vi "mtlb simx Call Script Function b.vi"(0 "clientID":i32, 1 "outString":string, 5 "variousIntsOut":i32, 7 "outInt":i32, 9 "outFloat":sgl, 11 "error in (no error)":errorcluster, 12 "outBuffer":string) -> (3 "outString out":string, 4 "function return":i32, 6 "variousIntsOut out":i32, 8 "outInt out":i32, 10 "outFloat out":sgl, 14 "outBuffer out":string, 15 "error out":errorcluster)   [LabVIEW 2019, in "PXL_V-REP.lvlib"]
doc: "EXTAPI_DLLEXPORT simxInt mtlb_simxCallScriptFunction_b(simxInt clientID,simxInt* variousIntsOut,simxInt** outInt,simxFloat** outFloat,simxChar** outString,simxUChar** outBuffer);"
uses:
  PXL_V-REP.lvlib
  <userlib>/V-REP/remoteApi.dll
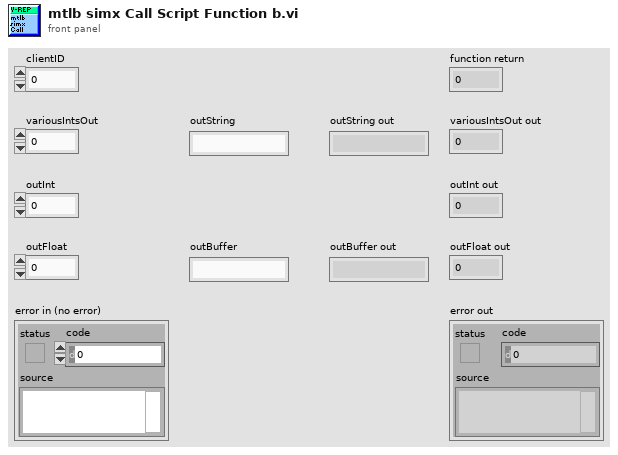
[diagram p1: front panel]
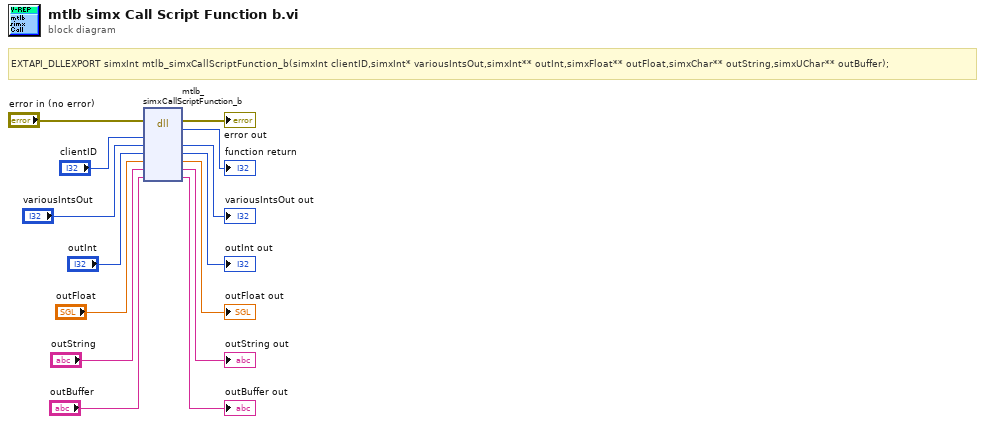
[diagram p0: block diagram]
diagram:
  # "EXTAPI_DLLEXPORT simxInt mtlb_simxCallScriptFunction_b(simxInt clientID,simxInt* variousIntsOut,simxInt** outInt,simxFloat** outFloat,simxChar** outString,simxUChar** outBuffer);"
  n1 = dll-call lib="C:/Program Files (x86)/National Instruments/LabVIEW 2019/user.lib/V-REP/remoteApi.*" fn="mtlb_simxCallScriptFunction_b"(error in="error in (no error)", "clientID"="clientID", "variousIntsOut"="variousIntsOut", "outInt"="outInt", "outFloat"="outFloat", "outString"="outString", "outBuffer"="outBuffer") -> (error out=→"error out":errorcluster, →"function return":i32, "variousIntsOut"=→"variousIntsOut out":i32, "outInt"=→"outInt out":i32, "outFloat"=→"outFloat out":sgl, "outString"=→"outString out":string, "outBuffer"=→"outBuffer out":string)  [unwired: 3 in, 1 out]
